vi "reprocess orientation.vi"(11 "file_in":string) -> (2 "function return":i32, 3 "file_in out":string)   [LabVIEW 2019, in "apdm.lvlib"]
doc: "APDM_EXPORT int apdm_reprocess_orientation(char *file_in);"
uses:
  apdm.lvlib
  Lee Lab/CP FES Walking 2018/Code/Working/LabVIEW/apdm.dll
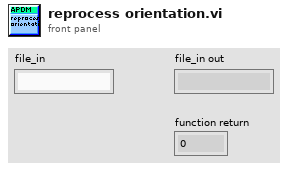
[diagram p1: front panel]
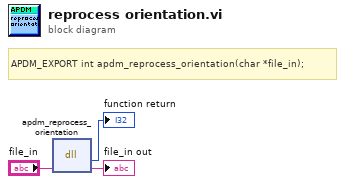
[diagram p0: block diagram]
diagram:
  # "APDM_EXPORT int apdm_reprocess_orientation(char *file_in);"
  n1 = dll-call lib="C:/Users/jfalesi/Dropbox/Lee Lab/CP FES Walking 2018/Code/Working/LabVIEW/apdm.*" fn="apdm_reprocess_orientation"("file_in"="file_in") -> (→"function return":i32, "file_in"=→"file_in out":string)  [unwired: 3 in, 2 out]
